vi "Protocol_Init.vi"(7 "Protocol":enum16{"RS-232", "TCP/IP", "Modbus TCP/IP"}(ring), 8 "error in (no error)":errorcluster, 10 "Com_Set":T1) -> (0 "error out":errorcluster, 3 "Protocol Out":refnum<class "Protocol.lvclass">)   [LabVIEW 2019, in "Protocol.lvclass"]
uses:
  Protocol.lvclass
  Modbus/Modbus.lvclass
  C:/Users/sesa588117/Desktop/SME_Client_App/04 Class/Protocol/Protocol.lvclass
  TCP/TCP.lvclass
  RS232/RS232.lvclass
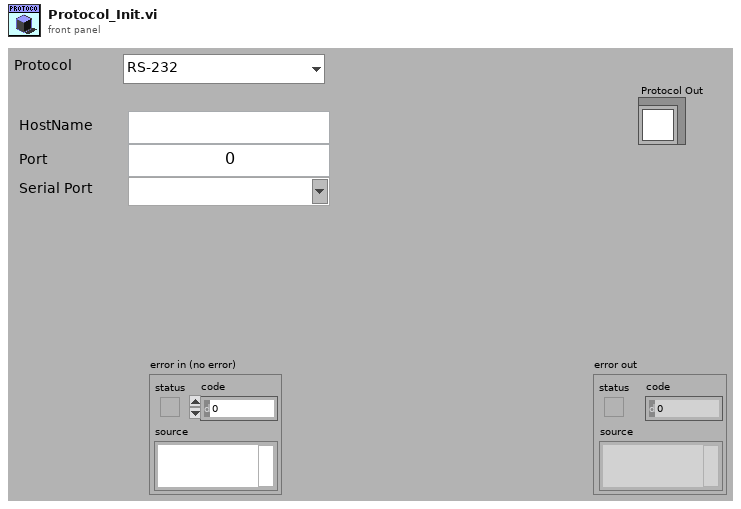
[diagram p1: front panel]
types:
  T1 = cluster{"HostName":string, "Port":u16, "ComPort":string}
  T2 = typedef "Modbus.lvclass/SettingCtrl.ctl" = cluster{"DevID":u16, "ComPort":string}
  T3 = typedef "TCP.lvclass/SettingCtrl.ctl" = cluster{"HostName":string, "Port":u16}
  T4 = typedef "RS232.lvclass/SettingCtrl.ctl" = cluster{"ComPort":string}
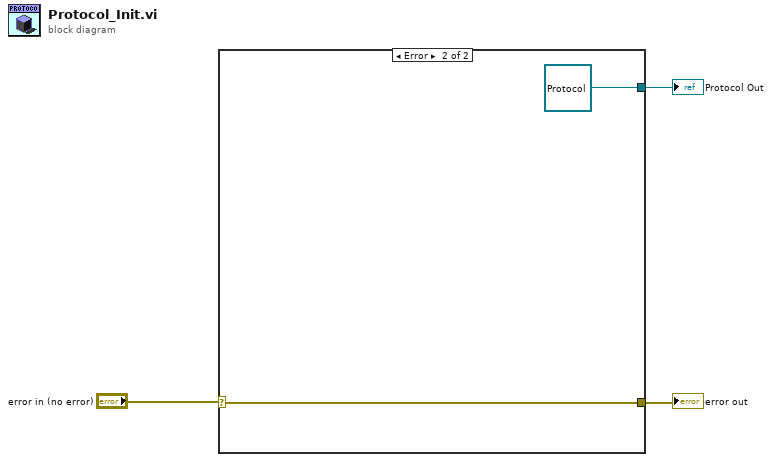
[diagram p0: block diagram]
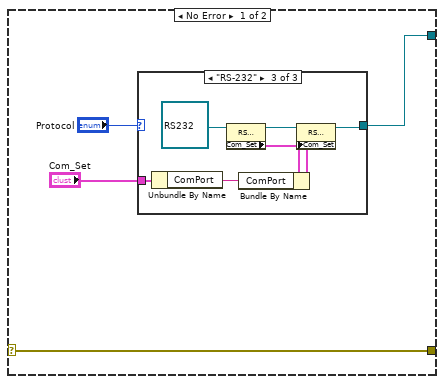
[diagram p2: hidden frame]
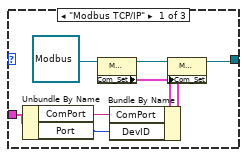
[diagram p3: hidden frame]
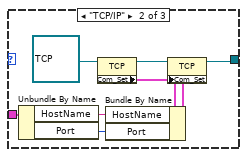
[diagram p4: hidden frame]
diagram:
  n1 = case shown="Error" "error in (no error)" {
    selector: "error in (no error)" -> [w7 w32]
    tunnel: [w6 refnum<class "Protocol.lvclass"> refnum ("Protocol")] -> w3
    tunnel: [w7 w32] -> w1
    frame No Error {
      n2 = case shown="\"RS-232\"" "Protocol" {
        tunnel: [w13 w21 w28] -> w6
        tunnel: "Com_Set" -> [w10 w18 w25]
        frame "Modbus TCP/IP" {
          n3 = Unbundle By Name(w10) -> ("ComPort"=w9:string, "Port"=w8:u16)
          n4 = property class="Modbus"(reference=refnum<class "Modbus.lvclass"> refnum ("Modbus")) -> (reference out=w14:refnum<class "Modbus.lvclass">, "Com_Set"=w12:T2)  [unwired: 1 in, 1 out]
          n5 = Bundle By Name(cluster=w12, "ComPort"=w9, "DevID"=w8) -> (w11:T2)
          n6 = property class="Modbus"(reference=w14, "Com_Set"=w11) -> (reference out=w13:refnum<class "Modbus.lvclass">)  [unwired: 1 in, 1 out]
        }
        frame "TCP/IP" {
          n7 = Unbundle By Name(w18) -> ("HostName"=w17:string, "Port"=w16:u16)
          n8 = property class="TCP"(reference=refnum<class "TCP.lvclass"> refnum ("TCP")) -> (reference out=w22:refnum<class "TCP.lvclass">, "Com_Set"=w20:T3)  [unwired: 1 in, 1 out]
          n9 = Bundle By Name(cluster=w20, "HostName"=w17, "Port"=w16) -> (w19:T3)
          n10 = property class="TCP"(reference=w22, "Com_Set"=w19) -> (reference out=w21:refnum<class "TCP.lvclass">)  [unwired: 1 in, 1 out]
        }
        frame "RS-232" {
          n11 = Unbundle By Name(w25) -> ("ComPort"=w24:string)
          n12 = property class="RS232"(reference=refnum<class "RS232.lvclass"> refnum ("RS232")) -> (reference out=w29:refnum<class "RS232.lvclass">, "Com_Set"=w27:T4)  [unwired: 1 in, 1 out]
          n13 = Bundle By Name(cluster=w27, "ComPort"=w24) -> (w26:T4)
          n14 = property class="RS232"(reference=w29, "Com_Set"=w26) -> (reference out=w28:refnum<class "RS232.lvclass">)  [unwired: 1 in, 1 out]
        }
      }
    }
    frame Error {
    }
  }
  "Protocol Out" <- w3
  "error out" <- w1
